vi "LakeShore VSM 7300 EMU.vi"(2 "Point #":i32, 3 "Instrument Address":refnum<visa-resource-name>) -> (0 "Stop":bool, 1 "Output":dbl[](array[numeric]) format="%.3e")   [LabVIEW 2021]
doc: "This VI reads the sample output of the Lakeshore DRC 93C or 82C temperature controller. The output is an array consisting of the single reading. The input is the numeric GPIB address.\nScott Hannahs, F. Bitter National Magnet Lab, 1993"
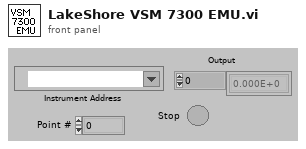
[diagram p1: front panel]
types:
  T1 = cluster{"Instrument":string, "ID Test String":string, "Terminator Character":string, u32, bool}
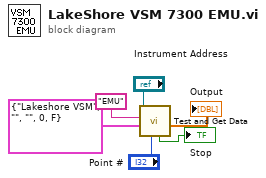
[diagram p0: block diagram]
diagram:
  n1 = call "Test and Get Data.vi"("Point #"="Point #", "Instrument Info"=T1 {"Instrument"="Lakeshore VSM", "ID Test String"="", "Terminator Character"="", 0, FALSE}, "Command String"="EMU", "VISA Sesson"="Instrument Address") -> ("Measurement"=→"Output":dbl[], "Stop"=→"Stop":bool)  [unwired: 2 in, 3 out]
